vi "P.vi"(8 "error in (no error)":errorcluster, 9 "Phi":dbl, 10 "Wire in":T1, 11 "Gate in":refnum<class "G-UE.lvclass">) -> (0 "error out":errorcluster, 3 "Gate out":refnum<class "G-UE.lvclass">)   [LabVIEW 2016, in "G-UE.lvclass"]
uses:
  G-UE.lvclass
  TypeDefs/Circuit Cluster.ctl
  GateAbst/GateAbst.lvclass
  <vilib>/Analysis/Matrix/Datatypes/ComplexMatrix.ctl
  <vilib>/Analysis/Matrix/NI_Matrix.lvlib
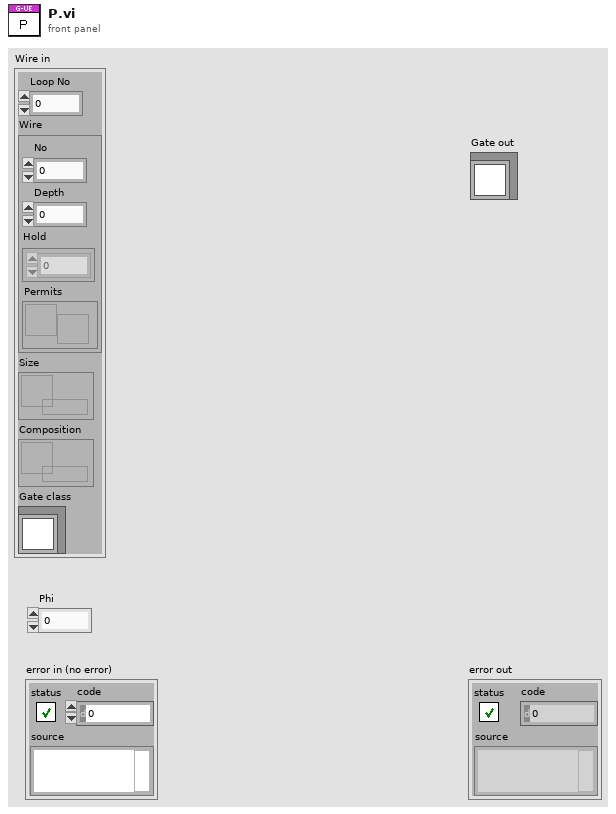
[diagram p1: front panel]
types:
  T1 = typedef "Circuit Cluster.ctl" = cluster{"Loop No":i32, "Wire":cluster{"No":i32, "Depth":i32, "Hold":i32[][], "Permits":refnum<notifier>}, "Size":refnum<queue>, "Composition":refnum<queue>, "Gate class":refnum<class "GateAbst.lvclass">}
  T2 = typedef "NI_Matrix.lvlib/ComplexMatrix.ctl" = cdb[][]
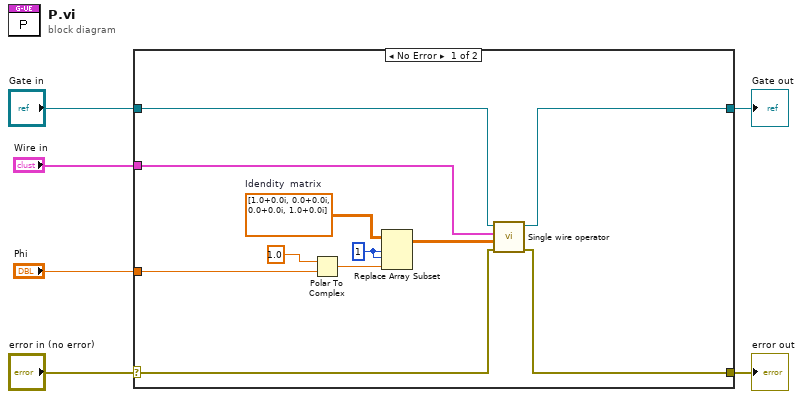
[diagram p0: block diagram]
diagram:
  n1 = case shown="No Error" "error in (no error)" {
    selector: "error in (no error)" -> [w14 w19]
    tunnel: [w15 w19] -> w5
    tunnel: [w16 w18] -> w3
    tunnel: "Gate in" -> [w17 w18]
    tunnel: "Phi" -> [w10 _]
    tunnel: "Wire in" -> [w13 _]
    frame No Error {
      w11 = 1 ("index (col)")
      w12 = T2 [[1.0+0.0i, 0.0+0.0i], [0.0+0.0i, 1.0+0.0i]]  # Idendity  matrix
      n2 = Polar To Complex(1:w10, 2:1.0 ("r")) -> (0:w8:cdb)
      n3 = Replace Array Subset ("Set Matrix Elements")(array=w12, new element=w8, index (row)=w11, index (col)=w11) -> (w7:T2)
      n4 = call "Single wire operator.vi"("error in (no error)"=w14, "Operator matrix"=w7, "Wire in"=w13, "G-UE in"=w17) -> ("error out"=w15:errorcluster, "G-UE out"=w16:refnum<class "G-UE.lvclass">)  [unwired: 6 in]
    }
    frame Error {
    }
  }
  "error out" <- w5
  "Gate out" <- w3
